vi "InitiateClientHandshake.vi"(4 "remote port or service name":u16=7890, 6 "address ('localhost')":string="localhost", 7 "additional headers (none)":T1[](array[typedef]), 8 "error in (no error)":errorcluster, 9 "timeout ms (5000)":i32=5000, 10 "request URI ('/')":string="/", 11 "TCP Connection in":refnum<k5>) -> (0 "error out":errorcluster, 2 "Server Headers Out":variant, 3 "WebSocket Client out":refnum<class "WebSocket Client.lvclass">)   [LabVIEW 2021, in "WebSockets.lvlib"]
doc: "**Deprecated - please use the new WebSocket.lvclass VIs instead. VI is retained for backwards compatibility.**\n\nPerforms a client-side handshake. Sends the initial handshake HTTP header and waits for response from WebSocket server. Validates received accept key from the response.\nWebSockets 2.0.1.40\nSam Sharp - MediaMongrels Ltd\nCopyright (c) 2019, MediaMongrels Ltd"
uses:
  WebSockets.lvlib
  WebSocket Client/WebSocket Client.lvclass
  D:/my_projects/projects/Algorithms/Labview/21/WebSockets/Source/WebSockets/WebSocket/WebSocket.lvclass
  WebSocket/Headers.ctl
  WebSocket/WebSocket.lvclass/WebSocket.ctl
  WebSocket/Read Return Headers.vi
  Sockets/VISA TCP Socket/VISA TCP.lvclass
  D:/my_projects/projects/Algorithms/Labview/21/WebSockets/Source/Sockets/Socket/Socket.lvclass
  WebSocket/Write Send Headers.vi
  WebSocket/WebSocket.lvclass
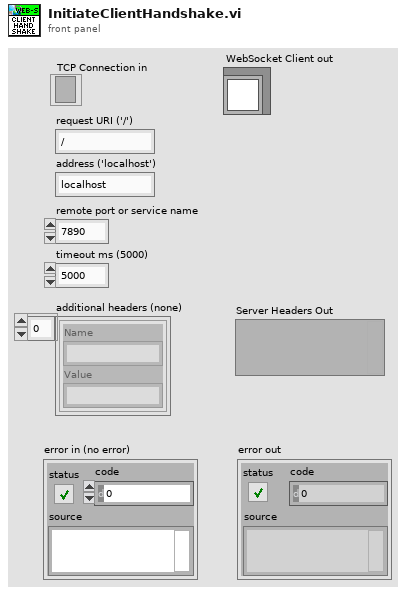
[diagram p1: front panel]
types:
  T1 = typedef "WebSockets.lvlib/WebSocket.lvclass/Headers.ctl" = cluster{"Name":string, "Value":string}
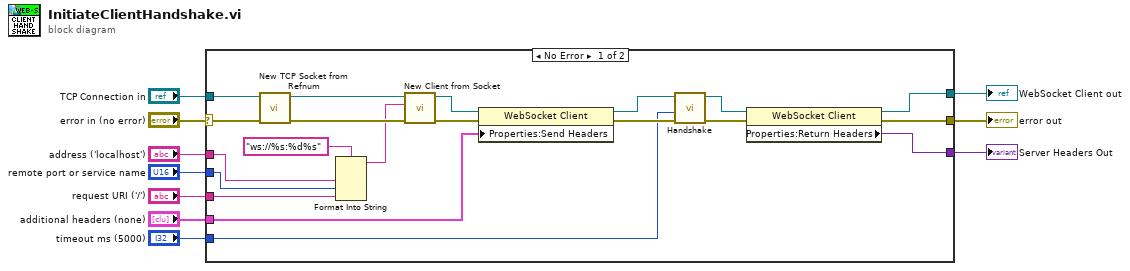
[diagram p0: block diagram]
diagram:
  n1 = case shown="No Error" "error in (no error)" {
    selector: "error in (no error)" -> [w17 w31]
    tunnel: [w19 _] -> w10
    tunnel: "TCP Connection in" -> [w16 _]
    tunnel: [w21 w31] -> w7
    tunnel: "timeout ms (5000)" -> [w26 _]
    tunnel: [w18 _] -> w5
    tunnel: "address ('localhost')" -> [w24 _]
    tunnel: "remote port or service name" -> [w23 _]
    tunnel: "additional headers (none)" -> [w30 _]
    tunnel: "request URI ('/')" -> [w22 _]
    frame No Error {
      n2 = call "New TCP Socket from Refnum.vi"("error in (no error)"=w17, "TCP Network Connection Refnum"=w16) -> ("error out"=w15:errorcluster, "VISA TCP out"=w14:refnum<class "VISA TCP.lvclass">)  [unwired: 8 in]
      n3 = Format Into String(format string="ws://%s:%d%s", w24, w23, w22) -> (resulting string=w11:string)  [unwired: 2 in, 1 out]
      n4 = call "New Client from Socket.vi"("error in (no error)"=w15, "WebSocket URL"=w11, "Socket in"=w14) -> ("error out"=w12:errorcluster, "WebSocket Client out"=w13:refnum<class "WebSocket Client.lvclass">)  [unwired: 7 in]
      n5 = property class="WebSocket Client"(reference=w13, error in=w12, "Properties:Send Headers"=w30) -> (reference out=w28:refnum<class "WebSocket Client.lvclass">, error out=w29:errorcluster)
      n6 = call-dynamic "Handshake.vi"("error in (no error)"=w29, "timeout ms (5000)"=w26, "WebSocket Client in"=w28) -> ("error out"=w27:errorcluster, "WebSocket Client out"=w20:refnum<class "WebSocket Client.lvclass">)  [unwired: 7 in]
      n7 = property class="WebSocket Client"(reference=w20, error in=w27) -> (reference out=w19:refnum<class "WebSocket Client.lvclass">, error out=w21:errorcluster, "Properties:Return Headers"=w18:variant)
    }
    frame Error {
    }
  }
  "WebSocket Client out" <- w10
  "error out" <- w7
  "Server Headers Out" <- w5
